vi "SSC Digital Write Source Waveform [Site Unique].vi"(0 "Digital SSC in":T1[](array[typedef]), 1 "Waveform Name":string, 5 "Per-Instrument Waveforms":u32[][][](array[numeric]) format="%.0x", 7 "Expand to Minimum Size?":bool caption="Expand to Minimum Size? (F)", 9 "Minimum Size":i32=128 caption="Minimum Size (128)", 11 "error in":errorcluster) -> (4 "Digital SSC out":T1[](array[typedef]), 15 "error out":errorcluster)   [LabVIEW 2020]
doc: "Writes one waveform per site after a waveform is created. Use this VI if you set the data mapping parameter of your source waveform to Site Unique."
uses:
  SSC Digital.ctl
  Shared SubVIs/Trim Whitespace [Inlined].vi
  <instrlib>/niDigital/niDigital.llb/niDigital Write Source Waveform (Site Unique U32).vi
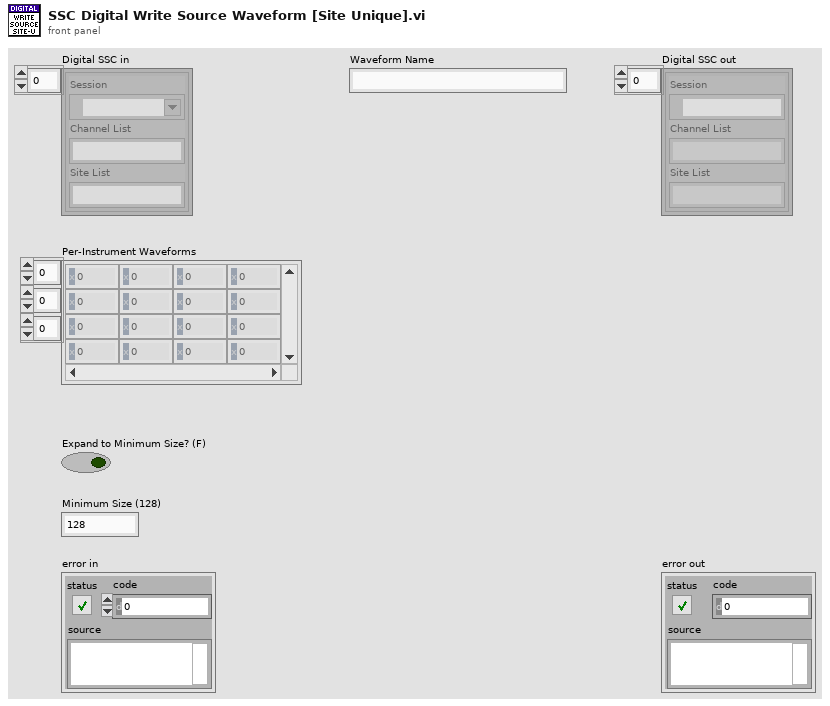
[diagram p1: front panel]
types:
  T1 = typedef "SSC Digital.ctl" = cluster{"Session":refnum<k15>, "Channel List":string, "Site List":string}
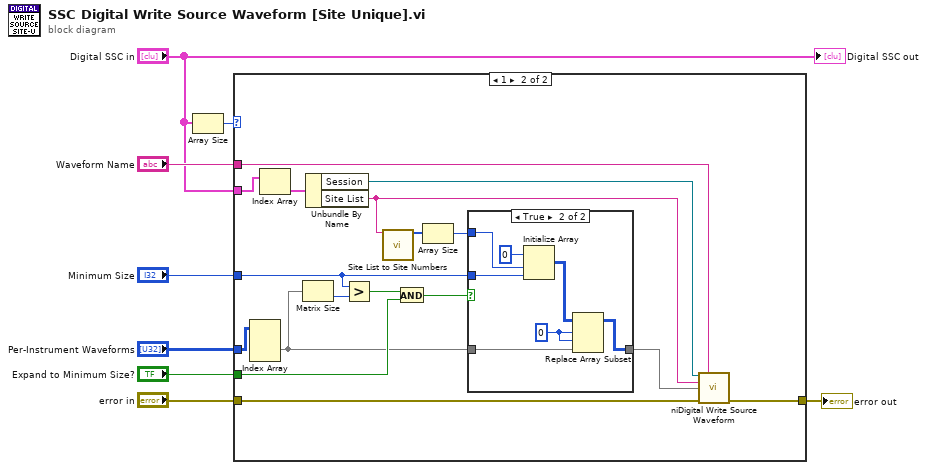
[diagram p0: block diagram]
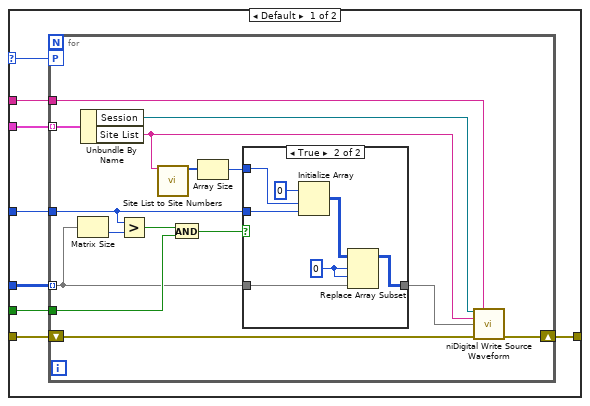
[diagram p2: hidden frame]
diagram:
  n1 = Array Size(array="Digital SSC in") -> (size(s)=w2:i32)
  n2 = case shown="1" w2 {
    selector: w2 -> [w10 _]
    tunnel: "Waveform Name" -> [w16 w56]
    tunnel: "error in" -> [w15 w55]
    tunnel: "Per-Instrument Waveforms" -> [w14 w54]
    tunnel: [w13 w53] -> w5
    tunnel: "Minimum Size" -> [w12 w52]
    tunnel: "Expand to Minimum Size?" -> [w11 w51]
    tunnel: "Digital SSC in" -> [w9 w50]
    frame Default {
      n3 = for {
        tunnel: w9 -> [w31] mode=indexing
        tunnel: w16 -> [w30]
        workers-P: w10 -> [_]
        tunnel: w14 -> [w22] mode=indexing
        shift-right: [w28] -> w13
        shift-left: w15 -> [w29]
        tunnel: w12 -> [w24]
        tunnel: w11 -> [w23]
        n4 = Matrix Size(0:w22) -> (2:w17:i32)  [unwired: 1 out]
        n5 = Unbundle By Name(w31) -> ("Session"=w27:refnum<k15>, "Site List"=w20:string)
        n6 = Greater?(x=w24, y=w17) -> (0:w26:bool)
        n7 = call "Site List to Site Numbers.vi"("Site List"=w20) -> ("Site Numbers"=w19:i32[])  [unwired: 13 in, 1 out]
        n8 = And(x=w26, y=w23) -> (x .and. y?=w25:bool)
        n9 = Array Size(array=w19) -> (size(s)=w18:i32)
        n10 = case shown="True" w25 {
          tunnel: w22 -> [w32 w37]
          tunnel: [w32 w36] -> w21
          tunnel: w24 -> [_ w33]
          tunnel: w18 -> [_ w34]
          frame False {
          }
          frame True {
            w35 = 0 ("index (row)")
            n11 = Initialize Array(u32 0 ("Numeric"), w34, w33) -> (w38:u32[][])
            n12 = Replace Array Subset(array=w38, new element=w37, index (row)=w35, index (col)=w35) -> (w36:u32[][])
          }
        }
        n13 = call-poly <instrlib>:"niDigital Write Source Waveform.vi"("instrument handle"=w27, "waveform name"=w30, "site list"=w20, "waveform data"=w21, "error in"=w29) -> ("error out"=w28:errorcluster)  [unwired: 9 in, 1 out]
      }
    }
    frame 1 {
      n14 = Index Array(array=w54) -> (element=w40:u32[][])  [unwired: 3 in]
      n15 = Index Array(array=w50) -> (element=w41:T1)  [unwired: 1 in]
      n16 = Matrix Size(0:w40) -> (2:w42:i32)  [unwired: 1 out]
      n17 = Unbundle By Name(w41) -> ("Session"=w49:refnum<k15>, "Site List"=w45:string)
      n18 = Greater?(x=w52, y=w42) -> (0:w48:bool)
      n19 = call "Site List to Site Numbers.vi"("Site List"=w45) -> ("Site Numbers"=w44:i32[])  [unwired: 13 in, 1 out]
      n20 = And(x=w48, y=w51) -> (x .and. y?=w47:bool)
      n21 = Array Size(array=w44) -> (size(s)=w43:i32)
      n22 = case shown="True" w47 {
        tunnel: w40 -> [w57 w62]
        tunnel: [w57 w61] -> w46
        tunnel: w52 -> [_ w58]
        tunnel: w43 -> [_ w59]
        frame False {
        }
        frame True {
          w60 = 0 ("index (row)")
          n23 = Initialize Array(u32 0 ("Numeric"), w59, w58) -> (w63:u32[][])
          n24 = Replace Array Subset(array=w63, new element=w62, index (row)=w60, index (col)=w60) -> (w61:u32[][])
        }
      }
      n25 = call-poly <instrlib>:"niDigital Write Source Waveform.vi"("instrument handle"=w49, "waveform name"=w56, "site list"=w45, "waveform data"=w46, "error in"=w55) -> ("error out"=w53:errorcluster)  [unwired: 9 in, 1 out]
    }
  }
  "error out" <- w5
  "Digital SSC out" <- "Digital SSC in"
